vi "LJM_eReadAddressArray.vi"(0 "Handle In":i32, 5 "Address":i32, 7 "Type":i32, 11 "error in":errorcluster, 13 "NumValues":i32) -> (4 "Handle Out":i32, 10 "aValues":dbl[](array[numeric]) format="%.2f", 14 "ErrorAddress":i32, 15 "error out":errorcluster)   [LabVIEW 2024]
uses:
  labjackm.dll
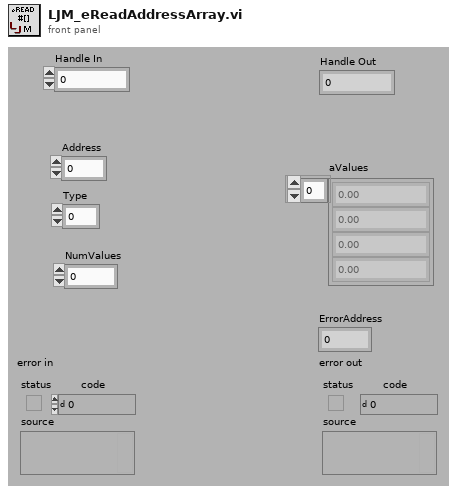
[diagram p1: front panel]
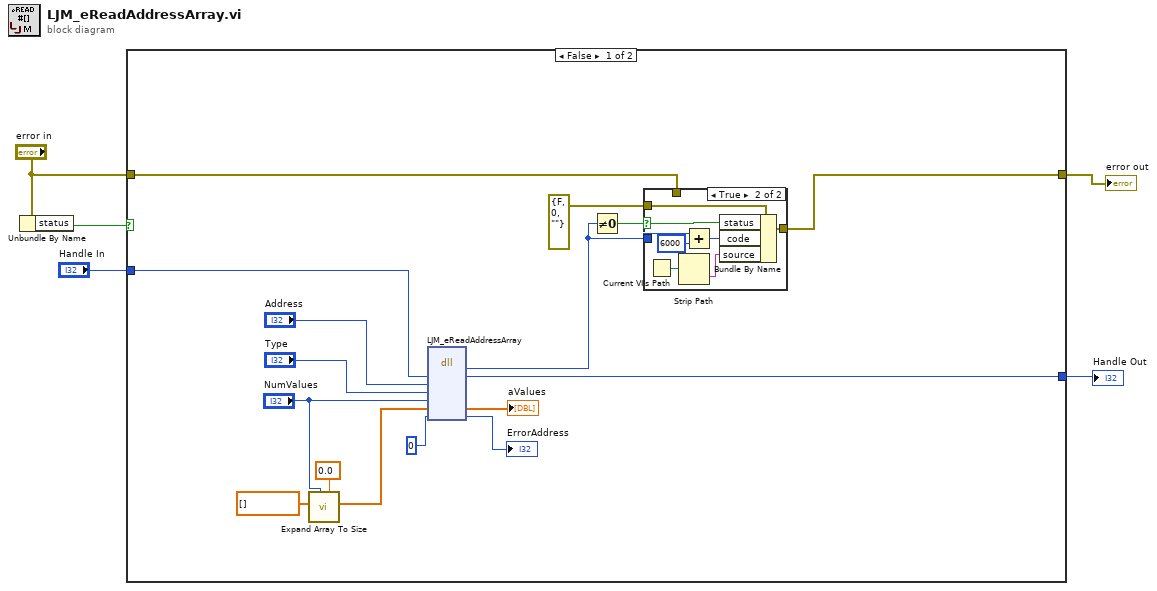
[diagram p0: block diagram]
diagram:
  n1 = Unbundle By Name("error in") -> ("status"=w5:bool)
  n2 = case shown="False" w5 {
    tunnel: "error in" -> [w18 w32]
    tunnel: [w17 w32] -> w3
    tunnel: [w10 w31] -> w2
    tunnel: "Handle In" -> [w9 w31]
    frame False {
      n3 = call "Expand Array To Size.vi"("Default Value"=0.0, "# Elements"="NumValues", "DBL Array In"=dbl[] []) -> ("DBL Array Out"=w14:dbl[])  [unwired: 4 in, 4 out]
      n4 = dll-call lib="labjackm.dll" fn="LJM_eReadAddressArray"("Handle"=w9, "Address"="Address", "Type"="Type", "NumValues"="NumValues", "aValues"=w14, "ErrorAddress"=u32 0 ("ErrorFrame")) -> (w21:i32, "Handle"=w10:i32, "aValues"=→"aValues":dbl[], "ErrorAddress"=→"ErrorAddress":i32)  [unwired: 6 in, 2 out]
      n5 = Not Equal To 0?(x=w21) -> (x != 0?=w20:bool)
      n6 = case shown="True" w20 {
        selector: w20 -> [_ w29]
        tunnel: [w22 w30] -> w17
        tunnel: errorcluster {"status"=FALSE, "code"=0, "source"=""} ("error IO") -> [_ w28]
        tunnel: w21 -> [_ w24]
        tunnel: w18 -> [w22 _]
        frame False {
        }
        frame True {
          n7 = Current VI's Path() -> (path=w26:path)
          n8 = Strip Path(path=w26) -> (name=w27:string)  [unwired: 1 out]
          n9 = Add(x=w24, y=6000) -> (x+y=w25:i32)
          n10 = Bundle By Name(cluster=w28, "status"=w29, "code"=w25, "source"=w27) -> (w30:errorcluster)
        }
      }
    }
    frame True {
    }
  }
  "error out" <- w3
  "Handle Out" <- w2
